vi "Get Application Version.vi"() -> (1 "run time system":bool, 2 "exe file last modification":timestamp, 3 "version number sentence":string, 4 "version number string":string)   [LabVIEW 2020, in "varilib.lvlib"]
doc: "Returns application version number and last modification date for compiled exe file. In the case of developement or other, returns describing text."
uses:
  varilib.lvlib
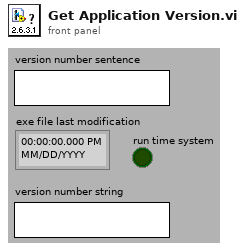
[diagram p1: front panel]
types:
  T1 = enum32{"invalid app kind", "Development System", "Run Time System", "Student Edition", "Embedded LabVIEW", "Evaluation", "Custom"}
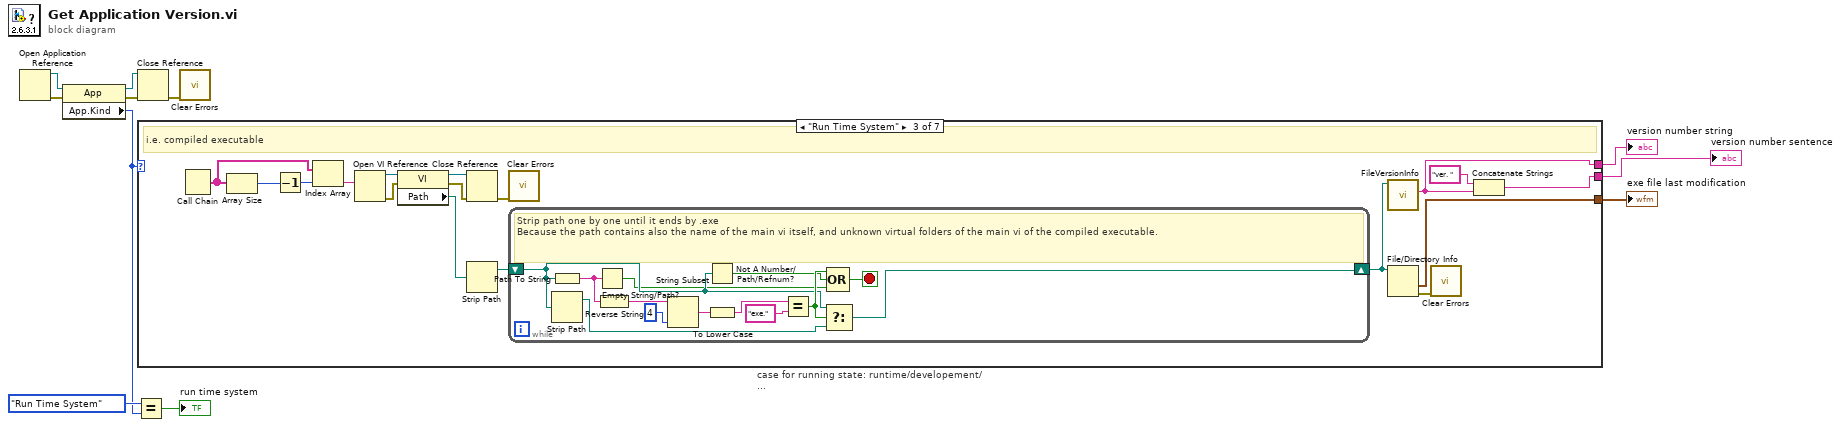
[diagram p0: block diagram]
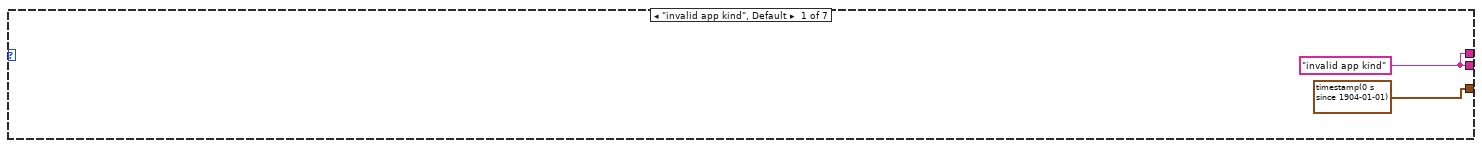
[diagram p2: hidden frame]
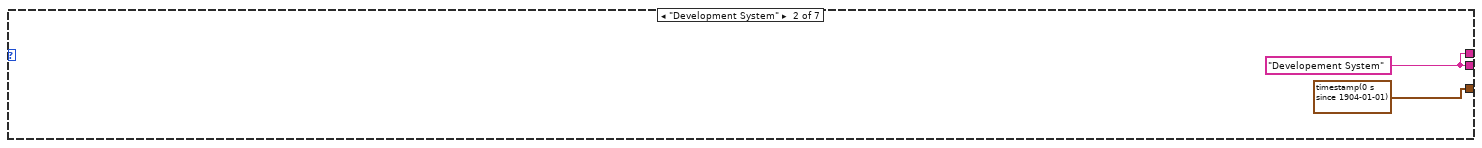
[diagram p3: hidden frame]
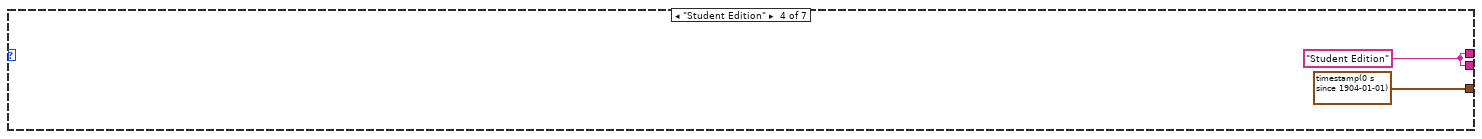
[diagram p4: hidden frame]
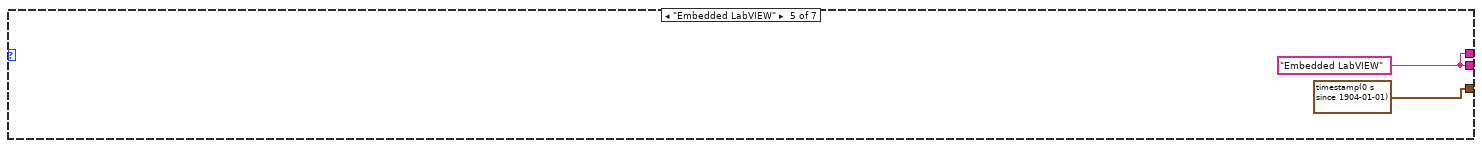
[diagram p5: hidden frame]
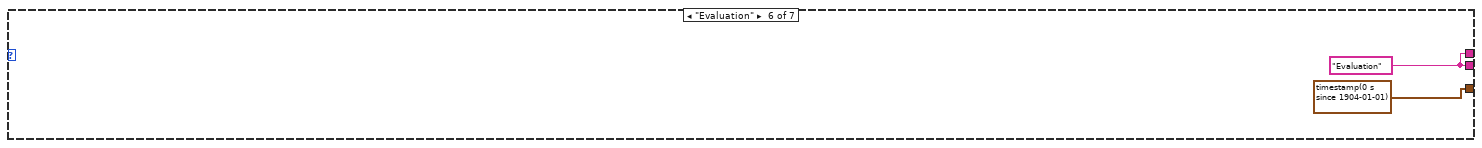
[diagram p6: hidden frame]
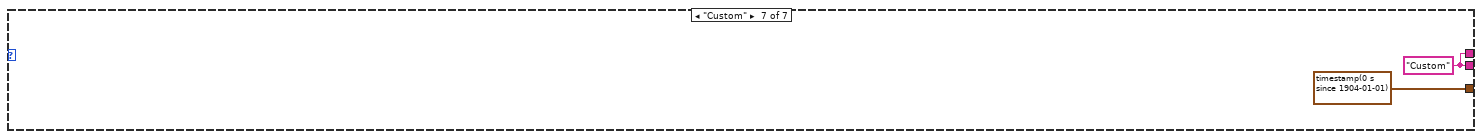
[diagram p7: hidden frame]
diagram:
  n1 = Open Application Reference() -> (0:w7:errorcluster, 3:w11:refnum<vi>)  [unwired: 4 in]
  n2 = property class="App"(reference=w11, error in=w7) -> (reference out=w5:refnum<vi>, error out=w6:errorcluster, "App.Kind"=w9:T1)
  n3 = Equal?(x=T1."Run Time System" ("Application:Kind"), y=w9) -> (x = y?=→"run time system":bool)
  n4 = Close Reference(reference=w5, error in (no error)=w6) -> (error out=w3:errorcluster)
  n5 = case "case for running state: runtime/developement/..." shown="\"Run Time System\"" w9 {
    tunnel: [w12 w14 w31 w46 w48 w50 w52] -> w2
    tunnel: [timestamp(0 s since 1904-01-01) ("last mod") timestamp(0 s since 1904-01-01) ("last mod") w21 timestamp(0 s since 1904-01-01) ("last mod") timestamp(0 s since 1904-01-01) ("last mod") timestamp(0 s since 1904-01-01) ("last mod") timestamp(0 s since 1904-01-01) ("last mod")] -> w4
    tunnel: [w12 w14 w18 w46 w48 w50 w52] -> w1
    frame "invalid app kind", Default {
      w12 = "invalid app kind"
    }
    frame "Development System" {
      w14 = "Developement System"
    }
    frame "Run Time System" {
      # "i.e. compiled executable"
      n6 = Call Chain() -> (call chain=w27:string[])
      n7 = Array Size(array=w27) -> (size(s)=w28:i32)
      n8 = Decrement(x=w28) -> (x-1=w26:i32)
      n9 = Index Array(array=w27, index=w26) -> (element=w25:string)
      n10 = Open VI Reference(vi path=w25) -> (vi reference=w29:refnum<vi>, error out=w30:errorcluster)  [unwired: 5 in]
      n11 = property class="VI"(reference=w29, error in=w30) -> (reference out=w23:refnum<vi>, error out=w24:errorcluster, "Path"=w22:path)
      n12 = Close Reference(reference=w23, error in (no error)=w24) -> (error out=w19:errorcluster)
      n13 = Strip Path(path=w22) -> (stripped path=w17:path)  [unwired: 1 out]
      n14 = call <vilib>:"Clear Errors.vi"("error in (no error)"=w19) -> ()  [unwired: 5 in, 2 out]
      n15 = while {
        shift-right: [w40] -> w16
        shift-left: w17 -> [w36]
        stop <- w37 stop-if-true
        # "Strip path one by one until it ends by .exe\nBecause the path contains also the name of the main vi itself, and unknown virtual folders of the main vi of the compiled executable."
        n16 = Path To String(path=w36) -> (string=w34:string)
        n17 = Strip Path(path=w36) -> (stripped path=w39:path)  [unwired: 1 out]
        n18 = Empty String/Path?(string/path=w34) -> (empty?=w33:bool)
        n19 = Reverse String(1:w34) -> (0:w45:string)
        n20 = String Subset(string=w45, length (rest)=4 ("length (rest)")) -> (substring=w42:string)  [unwired: 1 in]
        n21 = Not A Number/Path/Refnum?(number/path/refnum=w36) -> (NaN/Path/Refnum?=w35:bool)
        n22 = To Lower Case(string=w42) -> (all lower case string=w41:string)
        n23 = Equal?(x=w41, y="exe.") -> (x = y?=w38:bool)
        n24 = Select(t=w36, s=w38, f=w39) -> (s? t:f=w40:path)
        n25 = Compound Arithmetic op=OR(w38, w35, w33) -> (w37:bool)
      }
      n26 = call <vilib>:"FileVersionInfo.vi"("Application Path in"=w16) -> ("File Version Info"=w18:string)  [unwired: 7 in, 3 out]
      n27 = File/Directory Info(path=w16) -> (last mod=w21:timestamp, error out=w20:errorcluster)  [unwired: 1 in, 5 out]
      n28 = call <vilib>:"Clear Errors.vi"("error in (no error)"=w20) -> ()  [unwired: 5 in, 2 out]
      n29 = Concatenate Strings("ver. " ("string"), w18) -> (w31:string)
    }
    frame "Student Edition" {
      w46 = "Student Edition"
    }
    frame "Embedded LabVIEW" {
      w48 = "Embedded LabVIEW"
    }
    frame "Evaluation" {
      w50 = "Evaluation"
    }
    frame "Custom" {
      w52 = "Custom"
    }
  }
  "version number sentence" <- w2
  "exe file last modification" <- w4
  "version number string" <- w1
  n30 = call <vilib>:"Clear Errors.vi"("error in (no error)"=w3) -> ()  [unwired: 5 in, 2 out]
